vi "Render Polynomial in Picture.vi"(7 "origin":cluster{"x":i16, "y":i16}={"x"=20, "y"=20}, 9 "dependent variable":string="y", 10 "variable":string="x", 11 "coefficients":dbl[](array[numeric])) -> (3 "rendered equation":picture)   [LabVIEW 2023]
doc: "This VI renders a polynomial in a 2D Picture. This is used to improve visualization of polynomials."
uses:
  <vilib>/Analysis/polynomials.llb/Remove Zero Coefficients (DBL).vi
  <vilib>/Analysis/NI_AALPro.lvlib
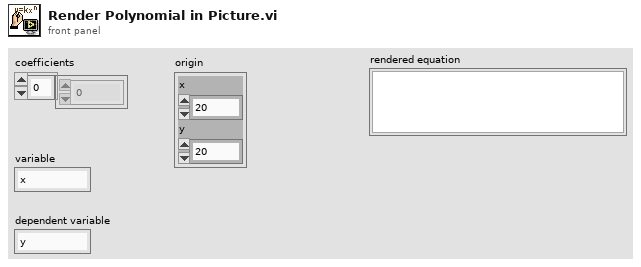
[diagram p1: front panel]
types:
  T1 = cluster{"horizontal":enum16{"left", "center", "right"}, "vertical":enum16{"top", "center", "bottom"}}
  T2 = cluster{"Font Name:":string, "Size":i16, "Strikeout?":bool, "Italic?":bool, "Underline?":bool, "Outline?":bool, "Shadow?":bool, "Bold?":bool}
  T3 = enum16{"User-specified Font", "Application Font", "System Font", "Dialog Font"}
  T4 = cluster{"left":i16, "top":i16, "right":i16, "bottom":i16}
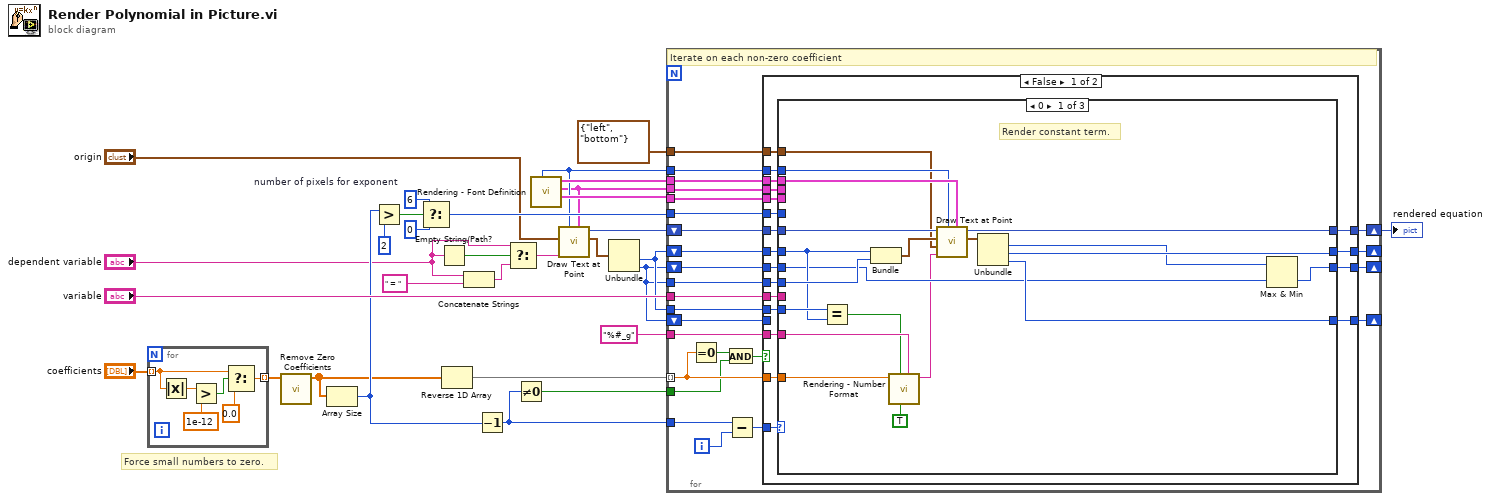
[diagram p0: block diagram]
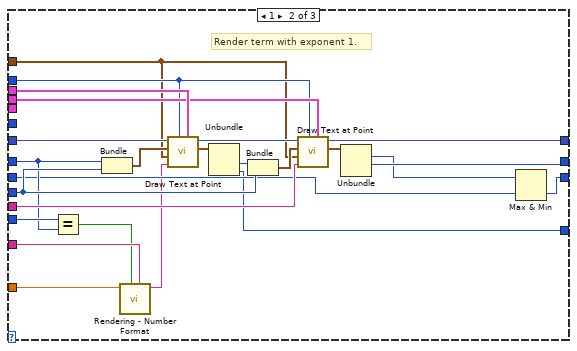
[diagram p2: hidden frame]
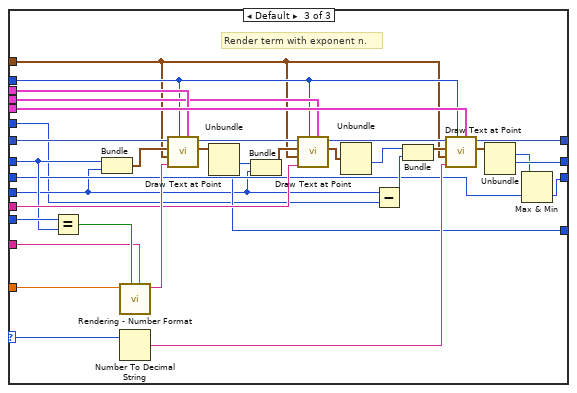
[diagram p3: hidden frame]
diagram:
  w26 = i16 6  # number of pixels for exponent
  # "Force small numbers to zero."
  n1 = for {
    tunnel: "coefficients" -> [w35] mode=indexing
    tunnel: [w34] -> w16 mode=indexing
    n2 = Absolute Value(x=w35) -> (abs(x)=w32:dbl)
    n3 = Greater?(x=w32, y=1e-12 ("tolerance")) -> (0:w36:bool)
    n4 = Select(t=w35, s=w36, f=0.0) -> (s? t:f=w34:dbl)
  }
  n5 = call-poly <vilib>:"Remove Zero Coefficients.vi"("P(x) In"=w16) -> ("P(x) Out"=w20:dbl[])  [unwired: 8 in, 2 out]
  n6 = Array Size(array=w20) -> (size(s)=w21:i32)
  n7 = Greater?(x=w21, y=2) -> (0:w2:bool)
  n8 = Select(t=w26, s=w2, f=i16 0) -> (s? t:f=w14:i16)
  n9 = Empty String/Path?(string/path="dependent variable") -> (empty?=w7:bool)
  n10 = Reverse 1D Array(array=w20) -> (reversed array=w29:dbl[])
  n11 = Concatenate Strings("dependent variable", " = " ("string")) -> (w9:string)
  n12 = Decrement(x=w21) -> (x-1=w23:i32)
  n13 = Select(t="dependent variable", s=w7, f=w9) -> (s? t:f=w8:string)
  n14 = Not Equal To 0?(x=w23) -> (x != 0?=w22:bool)
  n15 = call "Rendering - Font Definition.vi"() -> ("Exponent Font"=w19:T2, "Variable Font"=w5:T2, "Number Font"=w18:T2, "desired font(Application)"=w6:T3)  [unwired: 6 in, 2 out]
  n16 = call <vilib>:"Draw Text at Point.vi"("[user-specified font]"=w5, "desired font(Application)"=w6, "text"=w8, "origin"="origin") -> ("text rect"=w13:T4, "new picture"=w15:picture)  [unwired: 6 in]
  n17 = Unbundle(w13) -> ("right"=w12:i16, "bottom"=w11:i16)  [unwired: 2 out]
  n18 = for {
    tunnel: w29 -> [w42] mode=indexing
    shift-right: [w59] -> w24
    shift-left: w15 -> [w61]
    tunnel: "variable" -> [w60]
    shift-right: [w57] -> _
    shift-left: w12 -> [w58]
    tunnel: w11 -> [w56]
    tunnel: w18 -> [w55]
    tunnel: w19 -> [w54]
    tunnel: w5 -> [w53]
    tunnel: w12 -> [w52]
    tunnel: w23 -> [w50]
    shift-right: [w48] -> _
    shift-left: w11 -> [w49]
    tunnel: w6 -> [w47]
    shift-right: [w46] -> _
    shift-left: w11 -> [w45]
    tunnel: "%#_g" ("format string") -> [w44]
    tunnel: T1 {"horizontal"=enum."left", "vertical"=enum."bottom"} ("alignment(left, top)") -> [w43]
    tunnel: w14 -> [w40]
    tunnel: w22 -> [w38]
    i -> [w51]
    # "Iterate on each non-zero coefficient"
    n19 = Equal To 0?(x=w42) -> (x = 0?=w39:bool)
    n20 = And(x=w39, y=w38) -> (x .and. y?=w37:bool)
    n21 = Subtract(x=w50, y=w51) -> (x-y=w41:i32)
    n22 = case shown="False" w37 {
      tunnel: w61 -> [w80 w163]
      tunnel: w60 -> [w79 _]
      tunnel: [w78 w163] -> w59
      tunnel: w58 -> [w77 w162]
      tunnel: [w76 w162] -> w57
      tunnel: w42 -> [w75 _]
      tunnel: w56 -> [w74 _]
      tunnel: w55 -> [w73 _]
      tunnel: w54 -> [w72 _]
      tunnel: w53 -> [w71 _]
      tunnel: w52 -> [w70 _]
      tunnel: w41 -> [w69 _]
      tunnel: w49 -> [w68 w161]
      tunnel: [w67 w161] -> w48
      tunnel: w47 -> [w66 _]
      tunnel: [w65 w160] -> w46
      tunnel: w45 -> [_ w160]
      tunnel: w44 -> [w64 _]
      tunnel: w43 -> [w63 _]
      tunnel: w40 -> [w62 _]
      frame False {
        n23 = case shown="0" w69 {
          selector: w69 -> [_ _ w127]
          tunnel: w80 -> [w100 w125 w159]
          tunnel: w79 -> [_ w115 w141]
          tunnel: [w92 w112 w154] -> w78
          tunnel: w77 -> [w94 w113 w139]
          tunnel: [w93 w111 w137] -> w76
          tunnel: w75 -> [w83 w102 w129]
          tunnel: w74 -> [w96 w119 w128]
          tunnel: w73 -> [w97 w122 w150]
          tunnel: w72 -> [_ _ w151]
          tunnel: w71 -> [_ w117 w144]
          tunnel: w70 -> [w95 w114 w140]
          tunnel: w68 -> [w88 w110 w136]
          tunnel: [w86 w109 w134] -> w67
          tunnel: w66 -> [w91 w108 w133]
          tunnel: [w90 w107 w132] -> w65
          tunnel: w64 -> [w85 w104 w131]
          tunnel: w63 -> [w89 w106 w130]
          tunnel: w62 -> [_ _ w126]
          frame 0 {
            # "Render constant term."
            n24 = Equal?(x=w95, y=w94) -> (x = y?=w84:bool)
            n25 = Bundle("right"=w94, "bottom"=w96) -> (w98:cluster{"right":i16, "bottom":i16})  [unwired: 1 in]
            n26 = call "Rendering - Number Format.vi"("format string"=w85, "Is Lower Coefficient?"=TRUE, "Is Higher Coefficient?"=w84, "Coefficient"=w83) -> ("String Coefficient"=w82:string)  [unwired: 7 in]
            n27 = call <vilib>:"Draw Text at Point.vi"("[user-specified font]"=w97, "desired font(Application)"=w91, "text"=w82, "alignment(left, top)"=w89, "origin"=w98, "picture"=w100) -> ("text rect"=w99:T4, "new picture"=w92:picture)  [unwired: 4 in]
            n28 = Unbundle(w99) -> ("top"=w87:i16, "right"=w93:i16, "bottom"=w90:i16)  [unwired: 1 out]
            n29 = Max & Min(x=w87, y=w88) -> (min(x,y)=w86:i16)  [unwired: 1 out]
          }
          frame 1 {
            # "Render term with exponent 1."
            n30 = Equal?(x=w114, y=w113) -> (x = y?=w103:bool)
            n31 = Bundle("right"=w113, "bottom"=w119) -> (w123:cluster{"right":i16, "bottom":i16})  [unwired: 1 in]
            n32 = call "Rendering - Number Format.vi"("format string"=w104, "Is Higher Coefficient?"=w103, "Coefficient"=w102) -> ("String Coefficient"=w101:string)  [unwired: 8 in]
            n33 = call <vilib>:"Draw Text at Point.vi"("[user-specified font]"=w122, "desired font(Application)"=w108, "text"=w101, "alignment(left, top)"=w106, "origin"=w123, "picture"=w125) -> ("text rect"=w124:T4, "new picture"=w120:picture)  [unwired: 4 in]
            n34 = Unbundle(w124) -> ("right"=w116:i16, "bottom"=w107:i16)  [unwired: 2 out]
            n35 = Bundle("right"=w116, "bottom"=w119) -> (w121:cluster{"right":i16, "bottom":i16})  [unwired: 1 in]
            n36 = call <vilib>:"Draw Text at Point.vi"("[user-specified font]"=w117, "desired font(Application)"=w108, "text"=w115, "alignment(left, top)"=w106, "origin"=w121, "picture"=w120) -> ("text rect"=w118:T4, "new picture"=w112:picture)  [unwired: 4 in]
            n37 = Unbundle(w118) -> ("top"=w105:i16, "right"=w111:i16)  [unwired: 2 out]
            n38 = Max & Min(x=w105, y=w110) -> (min(x,y)=w109:i16)  [unwired: 1 out]
          }
          frame Default {
            # "Render term with exponent n."
            n39 = Equal?(x=w140, y=w139) -> (x = y?=w138:bool)
            n40 = Bundle("right"=w139, "bottom"=w128) -> (w156:cluster{"right":i16, "bottom":i16})  [unwired: 1 in]
            n41 = call "Rendering - Number Format.vi"("format string"=w131, "Is Higher Coefficient?"=w138, "Coefficient"=w129) -> ("String Coefficient"=w158:string)  [unwired: 8 in]
            n42 = Number To Decimal String(number=w127) -> (decimal integer string=w153:string)  [unwired: 1 in]
            n43 = call <vilib>:"Draw Text at Point.vi"("[user-specified font]"=w150, "desired font(Application)"=w133, "text"=w158, "alignment(left, top)"=w130, "origin"=w156, "picture"=w159) -> ("text rect"=w157:T4, "new picture"=w148:picture)  [unwired: 4 in]
            n44 = Unbundle(w157) -> ("right"=w143:i16, "bottom"=w132:i16)  [unwired: 2 out]
            n45 = Bundle("right"=w143, "bottom"=w128) -> (w149:cluster{"right":i16, "bottom":i16})  [unwired: 1 in]
            n46 = call <vilib>:"Draw Text at Point.vi"("[user-specified font]"=w144, "desired font(Application)"=w133, "text"=w141, "alignment(left, top)"=w130, "origin"=w149, "picture"=w148) -> ("text rect"=w146:T4, "new picture"=w147:picture)  [unwired: 4 in]
            n47 = Unbundle(w146) -> ("right"=w142:i16)  [unwired: 3 out]
            n48 = Subtract(x=w128, y=w126) -> (x-y=w152:i16)
            n49 = Bundle("right"=w142, w152) -> (w155:cluster{"right":i16, i16})  [unwired: 1 in]
            n50 = call <vilib>:"Draw Text at Point.vi"("[user-specified font]"=w151, "desired font(Application)"=w133, "text"=w153, "alignment(left, top)"=w130, "origin"=w155, "picture"=w147) -> ("text rect"=w145:T4, "new picture"=w154:picture)  [unwired: 4 in]
            n51 = Unbundle(w145) -> ("top"=w135:i16, "right"=w137:i16)  [unwired: 2 out]
            n52 = Max & Min(x=w135, y=w136) -> (min(x,y)=w134:i16)  [unwired: 1 out]
          }
        }
      }
      frame True {
        # "Do nothing is coefficient is zero."
      }
    }
  }
  "rendered equation" <- w24
